vi "Read Data in fF.vi"(8 "Error In":errorcluster, 11 "VISA IN":refnum<visa-resource-name>) -> (0 "Error Out":errorcluster, 1 "Output 2":string, 2 "Capacitance(fF)":string, 3 "VISA Out":refnum<visa-resource-name>, 4 "CAP (fF)":i32, 6 "Cap DBL":dbl)   [LabVIEW 2017]
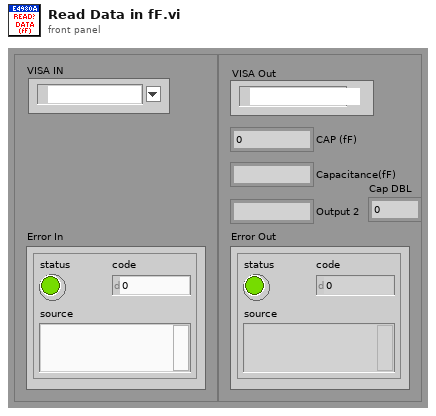
[diagram p1: front panel]
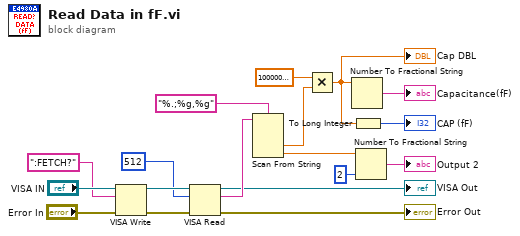
[diagram p0: block diagram]
diagram:
  n1 = VISA Write(VISA resource name="VISA IN", write buffer=":FETCH?", error in (no error)="Error In") -> (VISA resource name out=w15:refnum<visa-resource-name>, error out=w14:errorcluster)  [unwired: 1 out]
  n2 = VISA Read(VISA resource name=w15, byte count=u32 512, error in (no error)=w14) -> (VISA resource name out=→"VISA Out":refnum<visa-resource-name>, read buffer=w12:string, error out=→"Error Out":errorcluster)  [unwired: 1 out]
  n3 = Scan From String(format string="%.;%g,%g", input string=w12) -> (output 1=w8:dbl, output 2=w5:dbl)  [unwired: 4 in, 3 out]
  n4 = Multiply(x=1000000000000000.0, y=w8) -> (x*y=w1:dbl)
  "Cap DBL" <- w1
  n5 = Number To Fractional String(number=w1) -> (F-format string=→"Capacitance(fF)":string)  [unwired: 3 in]
  n6 = To Long Integer(number=w1) -> (32bit integer=→"CAP (fF)":i32)
  n7 = Number To Fractional String(number=w5, precision (6)=i16 2) -> (F-format string=→"Output 2":string)  [unwired: 2 in]
